vi "Wait for answer of longlasting command.vi"(0 "System no.":i32=1, 5 "error in":errorcluster, 12 "Stop refnum":refnum<vi>) -> (14 "Answer":bool, 15 "Stopped":bool, 19 "error out":errorcluster)   [LabVIEW 2026]
doc: "This VI waits for the answer of commands like REF, MPL, MNL or scanning routines using #7 polling and stops if answer has come, Stop refnum or Local stop is TRUE, or if a communications error occured. Sub-VI for long-lasting, one-axis commands and controller-algorithm commands. Requires #7.vi to be present. When using as a sub-VI, use Stop refnum to stop VI from caller."
uses:
  Communication/Global1.vi
panel:
  in  "Local stop":bool
  # "This vi waits for the answer of commands like REF, MPL, \nMNL or scanning routines using #7 polling and stops if \nanswer has come, Stop refnum or Local stop is TRUE, \nor if a communications error occured."
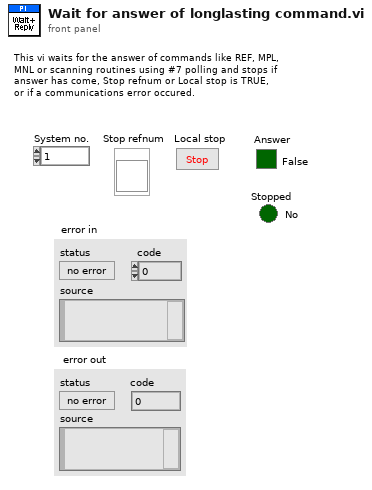
[diagram p1: front panel]
types:
  T1 = enum16{"Disable error check", "Force error check", "Use global settings"}
  T2 = typedef "Available interfaces.ctl" = u16
  T3 = cluster{"RS232 Portnumber":i32, "Timeout":i32, "RS232 Baud rate":u32, "Interface":T2, "GPIB Bus":i32, "GPIB Address":i32, "GPIB Mode":i32}[]
  T4 = cluster{"RS232 Portnumber":i32, "Timeout":i32, "RS232 Baud rate":u32, "Interface":T2, "GPIB Bus":i32, "GPIB Address":i32, "GPIB Mode":i32}
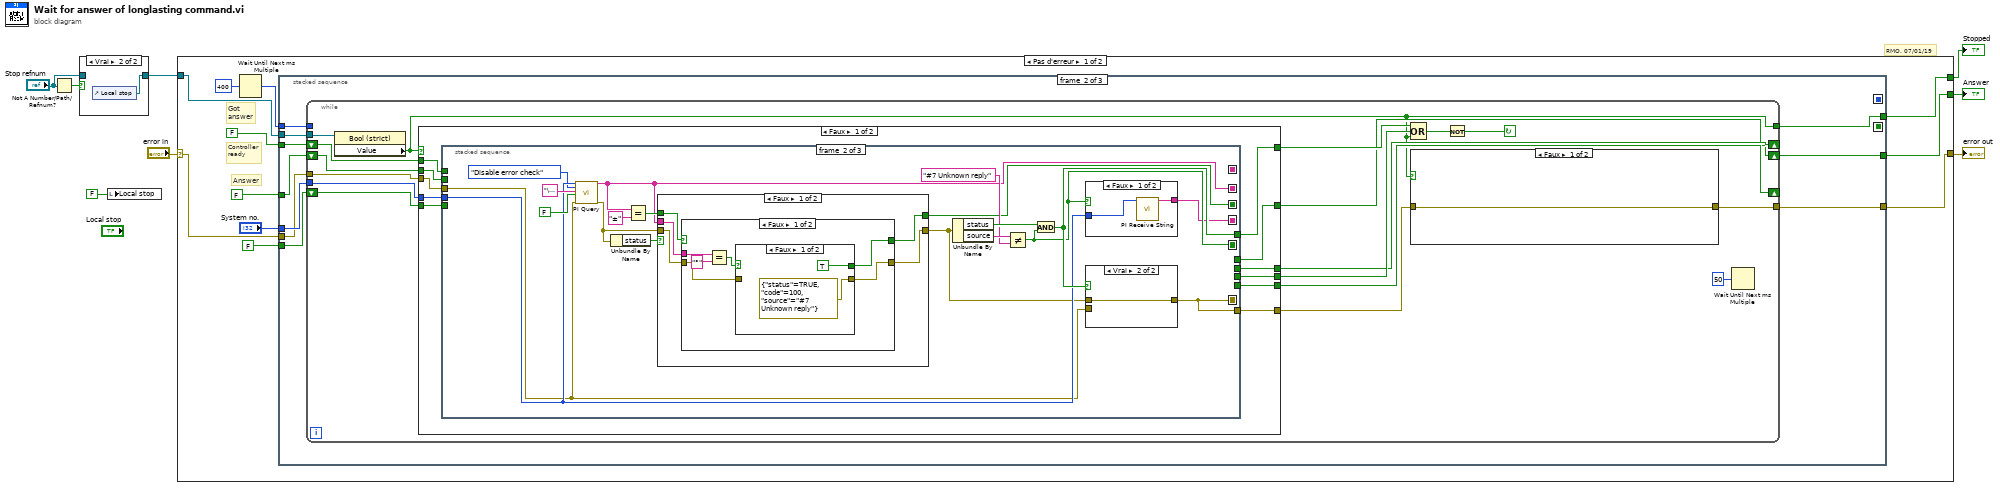
[diagram p0: block diagram]
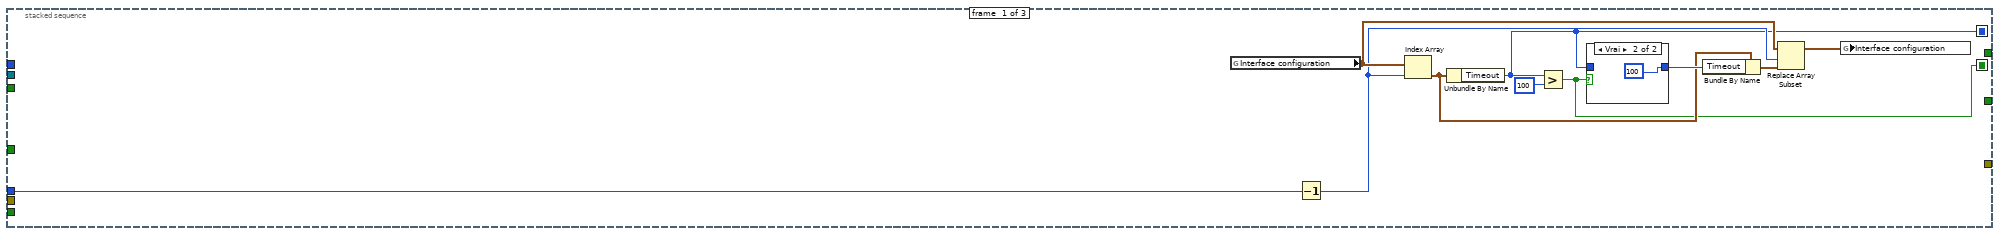
[diagram p3: hidden frame]
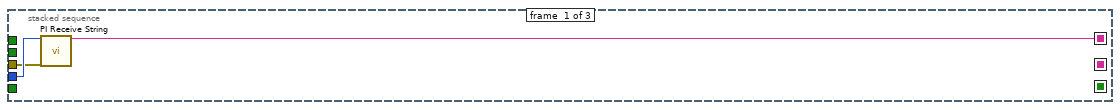
[diagram p5: hidden frame]
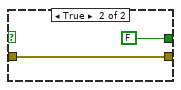
[diagram p6: hidden frame]
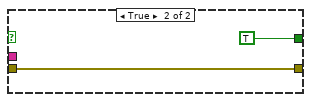
[diagram p7: hidden frame]
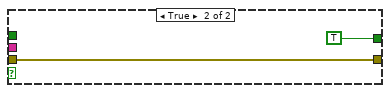
[diagram p8: hidden frame]
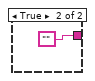
[diagram p9: hidden frame]
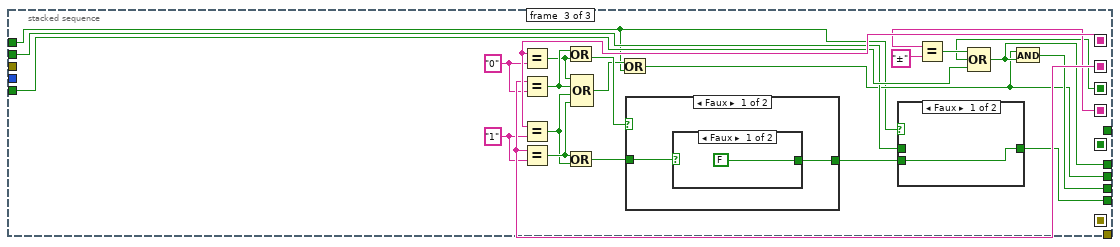
[diagram p11: hidden frame]
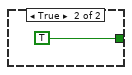
[diagram p13: hidden frame]
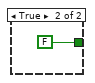
[diagram p14: hidden frame]
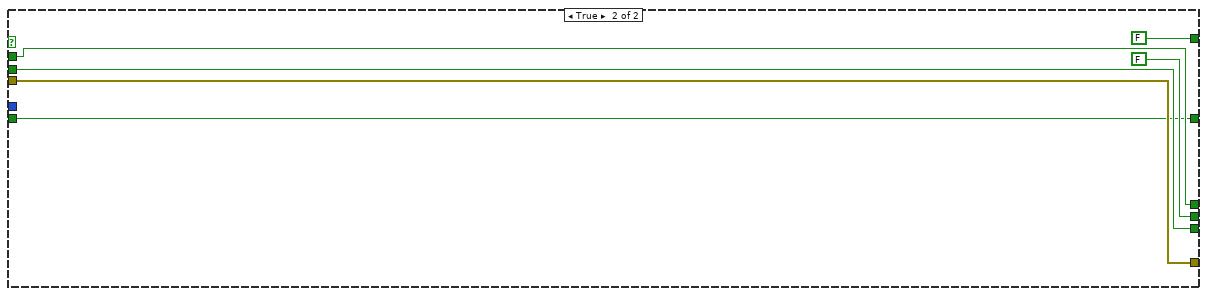
[diagram p15: hidden frame]
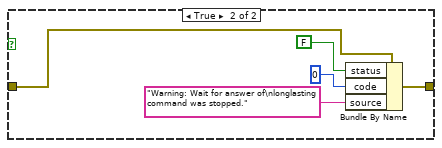
[diagram p16: hidden frame]
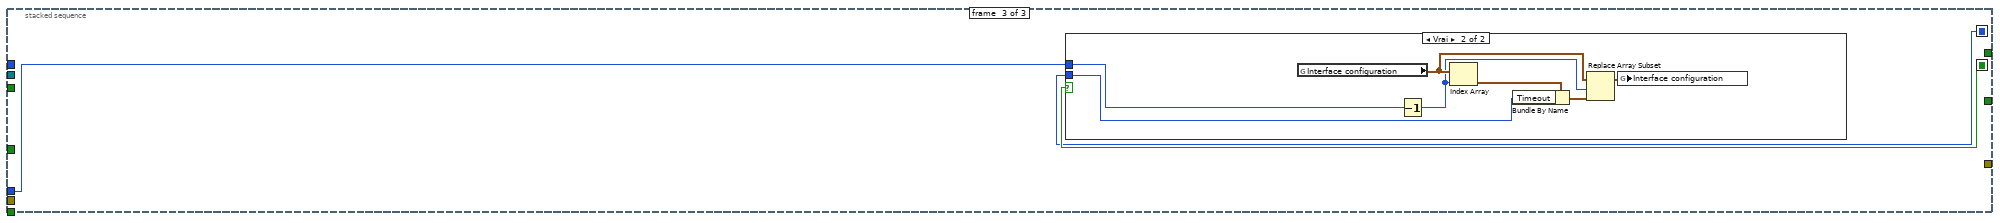
[diagram p17: hidden frame]
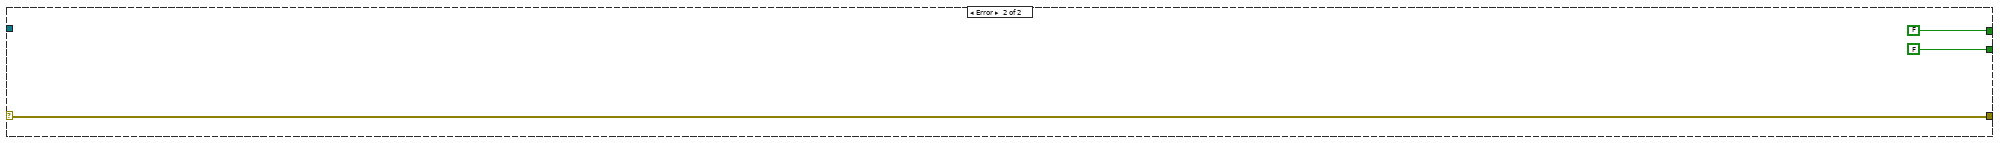
[diagram p19: hidden frame]
diagram:
  # "RMO, 07/01/19"
  n1 = Not A Number/Path/Refnum?(number/path/refnum="Stop refnum") -> (NaN/Path/Refnum?=w4:bool)
  n2 = case shown="Vrai" w4 {
    tunnel: [w9 w10] -> w2
    tunnel: "Stop refnum" -> [w9 _]
    frame False {
    }
    frame True {
      n3 = control-ref of="Local stop"() -> (w10:refnum<vi>)
    }
  }
  n4 = local write "Local stop"(FALSE ("Local stop")) -> ()
  n5 = case shown="Pas d'erreur" "error in" {
    selector: "error in" -> [w11 w170]
    tunnel: [w18 FALSE] -> w8
    tunnel: [w13 w170] -> w7
    tunnel: w2 -> [w14 _]
    tunnel: [w12 FALSE] -> w5
    frame No Error {
      # "Answer"
      # "Got\nanswer"
      # "Controller\nready"
      n6 = Wait Until Next ms Multiple(millisecond multiple=u32 400) -> (millisecond timer value=w15:u32)
      n7 = stacked-sequence {
        seq-local: [w23 _ _] -> [_ _ w160]
        seq-local: [w22 _ _] -> [_ _ w161]
        tunnel: "System no." -> [w28 w43 w162]
        tunnel: w11 -> [_ w42 _]
        tunnel: FALSE -> [_ w41 _]
        tunnel: FALSE -> [_ w40 _]
        tunnel: [_ w39 _] -> w18
        tunnel: FALSE -> [_ w38 _]
        tunnel: w15 -> [_ w37 _]
        tunnel: w14 -> [_ w36 _]
        tunnel: [_ w35 _] -> w13
        tunnel: [_ w34 _] -> w12
        frame #0 {
          n8 = global read "Global1.vi" "Interface configuration"() -> (w27:T3)
          n9 = Decrement(x=w28) -> (x-1=w25:i32)
          n10 = Index Array(array=w27, index=w25) -> (element=w29:T4)
          n11 = Unbundle By Name(w29) -> ("Timeout"=w23:i32)
          n12 = Greater?(x=w23, y=u32 100) -> (0:w22:bool)
          n13 = case shown="Vrai" w22 {
            tunnel: [w32 100] -> w30
            tunnel: w23 -> [w32 _]
            frame False {
            }
            frame True {
            }
          }
          n14 = Bundle By Name(cluster=w29, "Timeout"=w30) -> (w24:T4)
          n15 = Replace Array Subset(array=w27, new element=w24, index=w25) -> (w26:T3)
          n16 = global write "Global1.vi" "Interface configuration"(w26) -> ()
        }
        frame #1 {
          n17 = while {
            tunnel: [w44] -> w34
            tunnel: w36 -> [w45]
            tunnel: [w46] -> w35
            tunnel: w37 -> [_]
            shift-left: w38 -> [w48]
            shift-right: [w49] -> w39
            shift-left: w40 -> [w52]
            shift-right: [w53] -> _
            shift-left: w41 -> [w51]
            shift-right: [w50] -> _
            tunnel: w42 -> [w54]
            tunnel: w43 -> [w60]
            stop <- w57 continue-if-true
            n18 = property class="Bool (strict)"(reference=w45) -> ("Value"=w44:bool)  [unwired: 1 in, 2 out]
            n19 = case shown="Faux" w44 {
              tunnel: w60 -> [w71 _]
              tunnel: [w70 FALSE] -> w59
              tunnel: [w69 FALSE] -> w56
              tunnel: w54 -> [w68 w151]
              tunnel: [w67 w149] -> w53
              tunnel: w52 -> [w66 w149]
              tunnel: w51 -> [w65 w148]
              tunnel: [w64 w148] -> w50
              tunnel: [w63 w150] -> w49
              tunnel: w48 -> [w62 w150]
              tunnel: [w61 w151] -> w47
              frame False {
                n20 = stacked-sequence {
                  seq-local: [w74 _ _] -> [_ _ w140]
                  seq-local: [_ w76 _] -> [_ _ w133]
                  seq-local: [_ w87 _] -> [_ _ _]
                  seq-local: [_ w88 _] -> [_ _ w132]
                  seq-local: [_ w89 _] -> [_ _ _]
                  seq-local: [_ w79 _] -> [_ _ w129]
                  tunnel: w71 -> [w73 w81 _]
                  tunnel: [_ w90 _] -> w70
                  tunnel: [_ _ w126] -> w69
                  tunnel: w68 -> [w72 w80 _]
                  tunnel: [_ w87 _] -> w61
                  tunnel: [_ _ w122] -> w67
                  tunnel: w66 -> [_ _ w120]
                  tunnel: w65 -> [_ _ w128]
                  tunnel: [_ _ w127] -> w64
                  tunnel: [_ _ w125] -> w63
                  tunnel: w62 -> [_ _ w123]
                  frame #0 {
                    n21 = call "PI Receive String.vi"("System no."=w73, "error in"=w72) -> ("String read"=w74:string)  [unwired: 1 in, 16 out]
                  }
                  frame #1 {
                    n22 = call "PI Query.vi"("System no."=w81, "Error check settings"=T1."Disable error check", "String to send"="\u0007", "Attach termination char.?"=FALSE ("Attach Linefeed?"), "error in"=w80) -> ("String read"=w76:string, "error out"=w77:errorcluster)  [unwired: 2 in, 11 out]
                    n23 = Unbundle By Name(w77) -> ("status"=w85:bool)
                    n24 = Equal?(x=w76, y="±" ("String read")) -> (x = y?=w84:bool)
                    n25 = case shown="Faux" w85 {
                      tunnel: w84 -> [w98 _]
                      tunnel: [w97 w112] -> w78
                      tunnel: [w96 TRUE] -> w79
                      tunnel: w76 -> [w95 _]
                      tunnel: w77 -> [w94 w112]
                      frame False {
                        n26 = case shown="Faux" w98 {
                          tunnel: w94 -> [w101 w110]
                          tunnel: [w100 w110] -> w97
                          tunnel: [w102 TRUE] -> w96
                          tunnel: w95 -> [w104 _]
                          frame False {
                            n27 = Equal?(x=w104, y="°" ("String read")) -> (x = y?=w103:bool)
                            n28 = case shown="Faux" w103 {
                              tunnel: [TRUE FALSE] -> w102
                              tunnel: w101 -> [_ w107]
                              tunnel: [errorcluster {"status"=TRUE, "code"=100, "source"="#7 Unknown reply"} ("error out") w107] -> w100
                              frame False {
                              }
                              frame True {
                              }
                            }
                          }
                          frame True {
                          }
                        }
                      }
                      frame True {
                      }
                    }
                    n29 = Unbundle By Name(w78) -> ("status"=w93:bool, "source"=w92:string)
                    n30 = Not Equal?(x=w92, y="#7 Unknown reply" ("source")) -> (x != y?=w89:bool)
                    n31 = And(x=w93, y=w89) -> (x .and. y?=w90:bool)
                    n32 = case shown="Faux" w89 {
                      tunnel: w81 -> [w114 _]
                      tunnel: [w113 "" ("String read")] -> w88
                      frame False {
                        n33 = call "PI Receive String.vi"("System no."=w114) -> ("String read"=w113:string)  [unwired: 2 in, 16 out]
                      }
                      frame True {
                      }
                    }
                    n34 = case shown="Vrai" w90 {
                      tunnel: w78 -> [_ w117]
                      tunnel: [w116 w117] -> w87
                      tunnel: w80 -> [w116 _]
                      frame False {
                      }
                      frame True {
                      }
                    }
                  }
                  frame #2 {
                    w118 = "1"
                    w119 = "0"
                    n35 = Equal?(x=w140, y=w119) -> (x = y?=w138:bool)
                    n36 = Equal?(x=w133, y=w119) -> (x = y?=w139:bool)
                    n37 = Equal?(x=w140, y=w118) -> (x = y?=w135:bool)
                    n38 = Equal?(x=w133, y=w118) -> (x = y?=w136:bool)
                    n39 = Or(x=w139, y=w138) -> (x .or. y?=w137:bool)
                    n40 = Or(x=w136, y=w135) -> (x .or. y?=w134:bool)
                    n41 = Compound Arithmetic op=OR(w138, w139, w135, w136) -> (w121:bool)
                    n42 = Or(x=w121, y=w120) -> (x .or. y?=w122:bool)
                    n43 = case shown="Faux" w137 {
                      tunnel: [w144 FALSE] -> w124
                      tunnel: w134 -> [w143 _]
                      frame False {
                        n44 = case shown="Faux" w143 {
                          tunnel: [FALSE TRUE] -> w144
                          frame False {
                          }
                          frame True {
                          }
                        }
                      }
                      frame True {
                      }
                    }
                    n45 = case shown="Faux" w120 {
                      tunnel: [w141 w142] -> w125
                      tunnel: w124 -> [w141 _]
                      tunnel: w123 -> [_ w142]
                      frame False {
                      }
                      frame True {
                      }
                    }
                    n46 = Equal?(x=w132, y="±" ("String read")) -> (x = y?=w130:bool)
                    n47 = Compound Arithmetic op=OR(w130, w129, w128) -> (w127:bool)
                    n48 = And(x=w122, y=w127) -> (x .and. y?=w126:bool)
                  }
                }
              }
              frame True {
              }
            }
            n49 = Compound Arithmetic op=OR(w59, w56, w44) -> (w58:bool)
            n50 = case shown="Faux" w44 {
              tunnel: [w154 w158] -> w46
              tunnel: w47 -> [w154 w159]
              frame False {
              }
              frame True {
                n51 = Bundle By Name(cluster=w159, "status"=FALSE, "code"=0, "source"="Warning: Wait for answer of\nlonglasting command was stopped.") -> (w158:errorcluster)
              }
            }
            n52 = Not(x=w58) -> (.not. x?=w57:bool)
            n53 = Wait Until Next ms Multiple(millisecond multiple=u32 50) -> ()  [unwired: 1 out]
          }
        }
        frame #2 {
          n54 = case shown="Vrai" w161 {
            tunnel: w162 -> [_ w168]
            tunnel: w160 -> [_ w163]
            frame False {
            }
            frame True {
              n55 = global read "Global1.vi" "Interface configuration"() -> (w167:T3)
              n56 = Decrement(x=w168) -> (x-1=w165:i32)
              n57 = Index Array(array=w167, index=w165) -> (element=w169:T4)
              n58 = Bundle By Name(cluster=w169, "Timeout"=w163) -> (w164:T4)
              n59 = Replace Array Subset(array=w167, new element=w164, index=w165) -> (w166:T3)
              n60 = global write "Global1.vi" "Interface configuration"(w166) -> ()
            }
          }
        }
      }
    }
    frame Error {
    }
  }
  "Answer" <- w8
  "error out" <- w7
  "Stopped" <- w5
